vi "Constructor.vi"(8 "error in (no error)":errorcluster, 11 "Module Settings":T1) -> (0 "error out":errorcluster, 3 "Module.lvclass":refnum<class "Module.lvclass">)   [LabVIEW 2015, in "Module.lvclass"]
uses:
  Module.lvclass
  Module Settings.ctl
  IO/IO Class/Signal Settings.ctl
  Input Module/Input.lvclass
  Output Module/Output.lvclass
  Module.lvclass/Module.ctl
  IO/IO Class/IO Class.lvclass
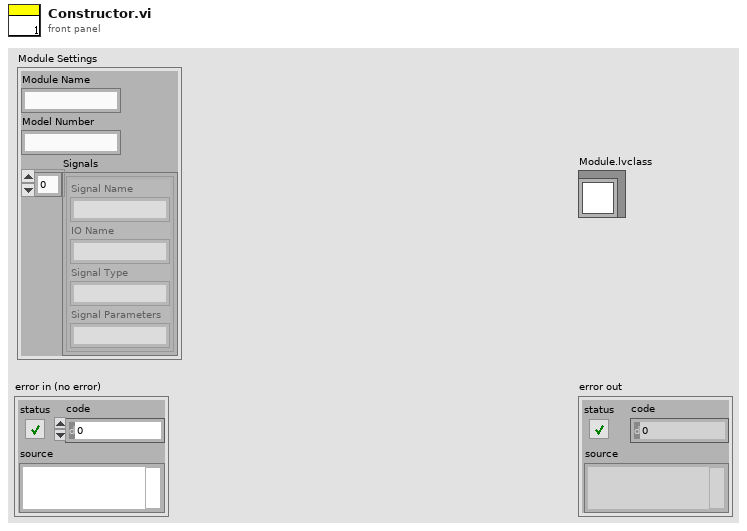
[diagram p1: front panel]
types:
  T1 = typedef "Module.lvclass/Module Settings.ctl" = cluster{"Module Name":string, "Model Number":string, "Signals":T2[]}
  T2 = typedef "IO Class.lvclass/Signal Settings.ctl" = cluster{"Signal Name":string, "IO Name":string, "Signal Type":string, "Signal Parameters":string}
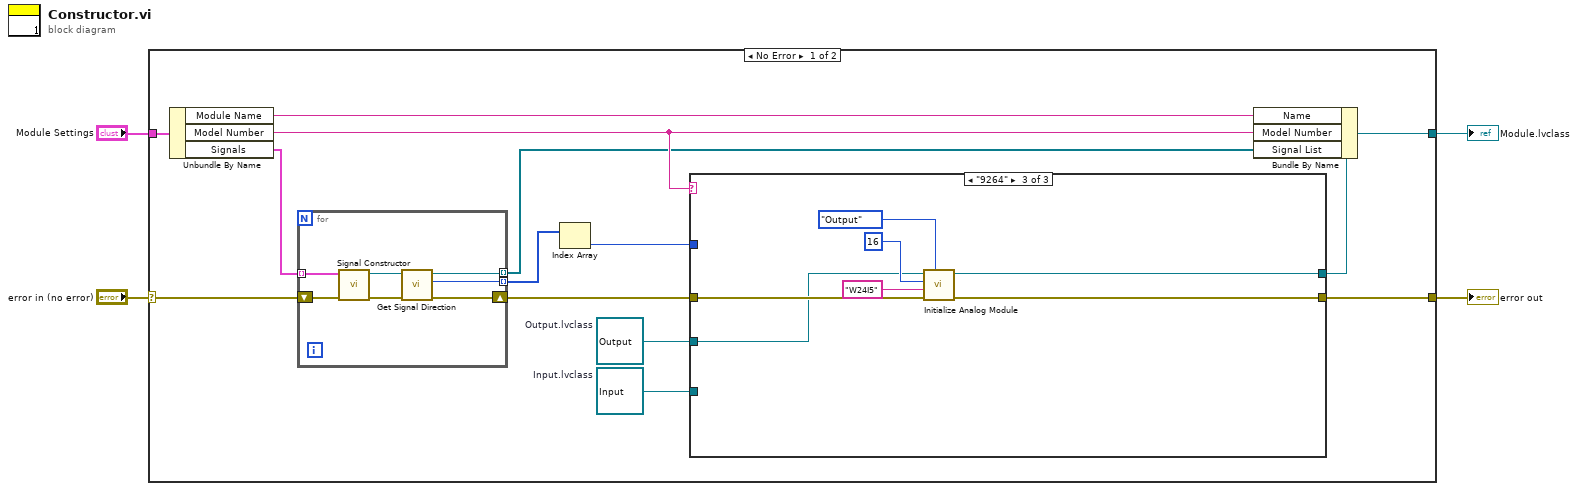
[diagram p0: block diagram]
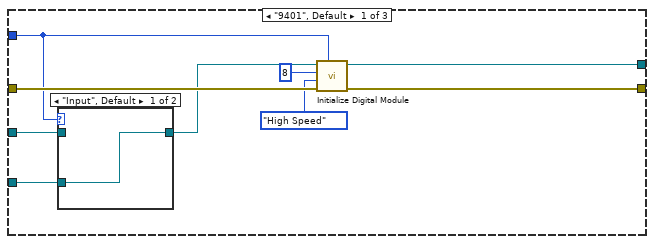
[diagram p2: hidden frame]
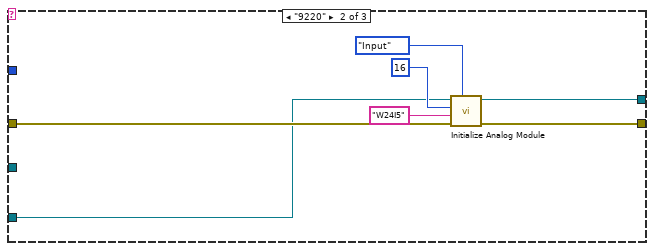
[diagram p4: hidden frame]
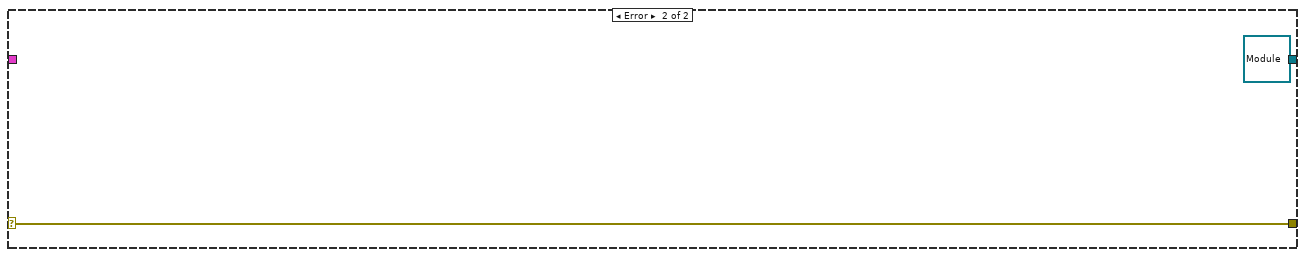
[diagram p5: hidden frame]
diagram:
  n1 = case shown="No Error" "error in (no error)" {
    selector: "error in (no error)" -> [w8 w52]
    tunnel: "Module Settings" -> [w17 _]
    tunnel: [w15 refnum<class "Module.lvclass"> refnum ("Module out")] -> w3
    tunnel: [w12 w52] -> w1
    frame No Error {
      w10 = refnum<class "Output.lvclass"> refnum  # Output.lvclass
      w11 = refnum<class "Input.lvclass"> refnum  # Input.lvclass
      n2 = Unbundle By Name(w17) -> ("Module Name"=w14:string, "Model Number"=w13:string, "Signals"=w9:T2[])
      n3 = for {
        tunnel: w9 -> [w50] mode=indexing
        shift-right: [w47] -> w5
        shift-left: w8 -> [w49]
        tunnel: [w45] -> w7 mode=indexing
        tunnel: [w44] -> w6 mode=indexing
        n4 = call "Signal Constructor.vi"("error in (no error)"=w49, "Signal Settings"=w50) -> ("error out"=w48:errorcluster, "IO Class.lvclass"=w46:refnum<class "IO Class.lvclass">)  [unwired: 8 in]
        n5 = call "Get Signal Direction.vi"("error in (no error)"=w48, "IO Class in"=w46) -> ("error out"=w47:errorcluster, "Direction"=w44:enum16{"Input", "Output"}, "IO Class out"=w45:refnum<class "IO Class.lvclass">)  [unwired: 7 in]
      }
      n6 = Index Array(array=w6) -> (element=w18:enum16{"Input", "Output"})  [unwired: 1 in]
      n7 = case shown="\"9264\"" w13 {
        tunnel: [w27 w36 w43] -> w16
        tunnel: w5 -> [w26 w31 w42]
        tunnel: [w25 w35 w41] -> w12
        tunnel: w18 -> [w22 _ _]
        tunnel: w11 -> [w20 w30 _]
        tunnel: w10 -> [w21 _ w37]
        frame "9401", Default {
          n8 = case shown="\"Input\", Default" w22 {
            tunnel: w21 -> [_ w29]
            tunnel: w20 -> [w28 _]
            tunnel: [w28 w29] -> w19
            frame "Input", Default {
            }
            frame "Output" {
            }
          }
          n9 = call "Initialize Digital Module.vi"("Direction"=w22, "error in (no error)"=w26, "Speed"=enum16{"High Speed", "Low Speed"}."High Speed", "Channels"=u8 8, "Module in"=w19) -> ("error out"=w25:errorcluster, "Module out"=w27:refnum<class "Module.lvclass">)  [unwired: 5 in]
        }
        frame "9220" {
          n10 = call "Initialize Analog Module.vi"("Direction"=enum16{"Input", "Output"}."Input", "error in (no error)"=w31, "FXP Type"="W24I5", "Channels"=u8 16, "Module in"=w30) -> ("error out"=w35:errorcluster, "Module out"=w36:refnum<class "Input.lvclass">)  [unwired: 5 in]
        }
        frame "9264" {
          n11 = call "Initialize Analog Module.vi"("Direction"=enum16{"Input", "Output"}."Output", "error in (no error)"=w42, "FXP Type"="W24I5", "Channels"=u8 16, "Module in"=w37) -> ("error out"=w41:errorcluster, "Module out"=w43:refnum<class "Output.lvclass">)  [unwired: 5 in]
        }
      }
      n12 = Bundle By Name(cluster=w16, "Name"=w14, "Model Number"=w13, "Signal List"=w7) -> (w15:refnum<class "Module.lvclass">)
    }
    frame Error {
    }
  }
  "Module.lvclass" <- w3
  "error out" <- w1
